vi "Init.vi"(8 "error in":errorcluster, 11 "NEO480 in":refnum<class "Virtual NEO480.lvclass">) -> (0 "error out":errorcluster, 3 "NEO480 out":refnum<class "Virtual NEO480.lvclass">)   [LabVIEW 2024, in "Virtual NEO480.lvclass"]
uses:
  Virtual NEO480.lvclass
  Virtual NEO480.lvclass/Virtual NEO480.ctl
  Source/Interfaces/IConfiguration/IConfiguration.lvclass
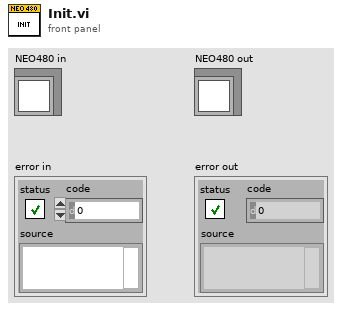
[diagram p1: front panel]
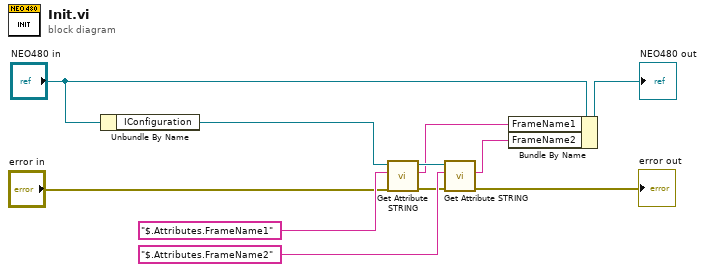
[diagram p0: block diagram]
diagram:
  n1 = Unbundle By Name("NEO480 in") -> ("IConfiguration"=w11:refnum<class "IConfiguration.lvclass">)
  n2 = call-dynamic "Get Attribute STRING.vi"("error in"="error in", "Attribute"="$.Attributes.FrameName1", "IConfiguration in"=w11) -> ("error out"=w5:errorcluster, "Value"=w3:string, "IConfiguration out"=w8:refnum<class "IConfiguration.lvclass">)  [unwired: 6 in]
  n3 = call-dynamic "Get Attribute STRING.vi"("error in"=w5, "Attribute"="$.Attributes.FrameName2", "IConfiguration in"=w8) -> ("error out"=→"error out":errorcluster, "Value"=w2:string)  [unwired: 6 in, 1 out]
  n4 = Bundle By Name(cluster="NEO480 in", "FrameName1"=w3, "FrameName2"=w2) -> (→"NEO480 out":refnum<class "Virtual NEO480.lvclass">)
